vi "Read Double.vi"(8 "error in (no error)":errorcluster, 11 "DataSingleElement in":refnum<class "DataSingleElement.lvclass">) -> (0 "error out":errorcluster, 2 "value":dbl, 3 "DataSingleElement out":refnum<class "DataSingleElement.lvclass">)   [LabVIEW 2014, in "DataSingleElement.lvclass"]
uses:
  DataSingleElement.lvclass
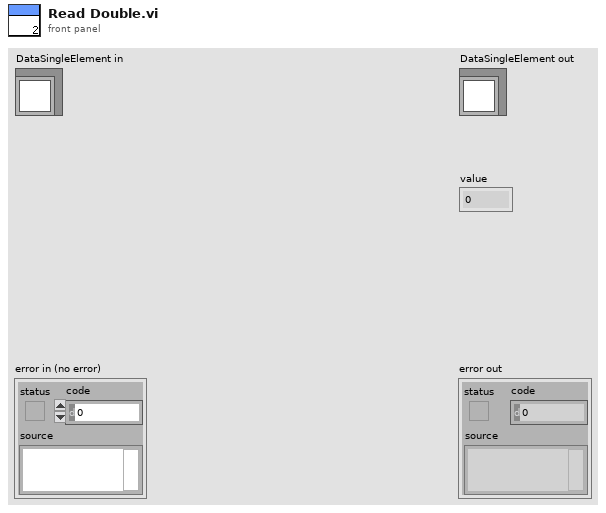
[diagram p1: front panel]
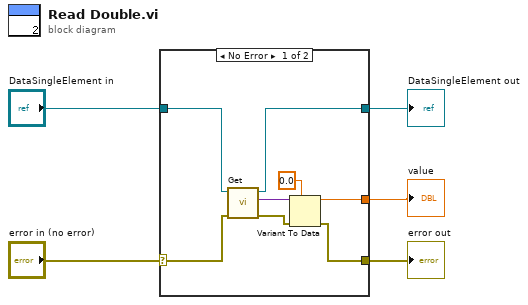
[diagram p0: block diagram]
diagram:
  n1 = case shown="No Error" "error in (no error)" {
    selector: "error in (no error)" -> [w13 w15]
    tunnel: [w7 w15] -> w4
    tunnel: [w10 w14] -> w2
    tunnel: "DataSingleElement in" -> [w11 w14]
    tunnel: [w6 _] -> w1
    frame No Error {
      n2 = call-dynamic "Get.vi"("error in (no error)"=w13, "AbstractData in"=w11) -> ("error out"=w8:errorcluster, "Data"=w12:variant, "AbstractData out"=w10:refnum<class "DataSingleElement.lvclass">)  [unwired: 7 in]
      n3 = Variant To Data(error in=w8, type=0.0, Variant=w12) -> (data=w6:dbl, error out=w7:errorcluster)
    }
    frame Error {
    }
  }
  "error out" <- w4
  "DataSingleElement out" <- w2
  "value" <- w1
